vi "Validate Path.vi"(11 "Path in":path) -> (3 "Path out":path)   [LabVIEW 2019, in "Panel.lvlib" / "Persistent Position.lvclass"]
doc: "Checks a path for validity. If the input path is not valid, a default valid path will be generated.\n\n----\nPlease see the following web address for additional documentation and tutorial information:\nhttp://www.mooregoodideas.com/mgi-panel-manager/\n\nAuthor: Derek Trepanier\n\nCopyright (c) 2018, Moore Good Ideas, Inc.\n\nAll rights reserved.\n\nRedistribution and use in source and binary forms, with or without modification, are permitted provided that the following conditions are met:\n\n * Redistributions of source code must retain the above copyright notice, this list of conditions and the following disclaimer.\n * Redistributions in binary form must reproduce the above copyright notice, this list of conditions and the following disclaimer in the documentation and/or other materials provided with the distribution.\n * Neither the name of Moore Good Ideas, Inc. nor the names of its contributors may be used to endorse or promote products derived from this software without specific prior written permission.\n\nTHIS SOFTWARE IS PROVIDED BY THE COPYRIGHT HOLDERS AND CONTRIBUTORS \"AS IS\" AND ANY EXPRESS OR IMPLIED WARRANTIES, INCLUDING, BUT NOT LIMITED TO, THE IMPLIED WARRANTIES OF MERCHANTABILITY AND FITNESS FOR A PARTICULAR PURPOSE ARE DISCLAIMED. IN NO EVENT SHALL THE COPYRIGHT OWNER OR CONTRIBUTORS BE LIABLE FOR ANY DIRECT, INDIRECT, INCIDENTAL, SPECIAL, EXEMPLARY, OR CONSEQUENTIAL DAMAGES (INCLUDING, BUT NOT LIMITED TO, PROCUREMENT OF SUBSTITUTE GOODS OR SERVICES; LOSS OF USE, DATA, OR PROFITS; OR BUSINESS INTERRUPTION) HOWEVER CAUSED AND ON ANY THEORY OF LIABILITY, WHETHER IN CONTRACT, STRICT LIABILITY, OR TORT (INCLUDING NEGLIGENCE OR OTHERWISE) ARISING IN ANY WAY OUT OF THE USE OF THIS SOFTWARE, EVEN IF ADVISED OF THE POSSIBILITY OF SUCH DAMAGE."
uses:
  Persistent Position.lvclass
  <vilib>/Utility/sysdir.llb/System Directory Type.ctl
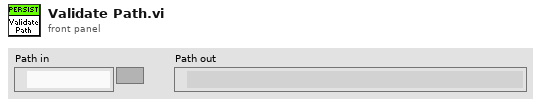
[diagram p1: front panel]
types:
  T1 = typedef "System Directory Type.ctl" = i32
  T2 = enum32{"invalid app kind", "Development System", "Run Time System", "Student Edition", "Embedded LabVIEW", "Evaluation", "Custom"}
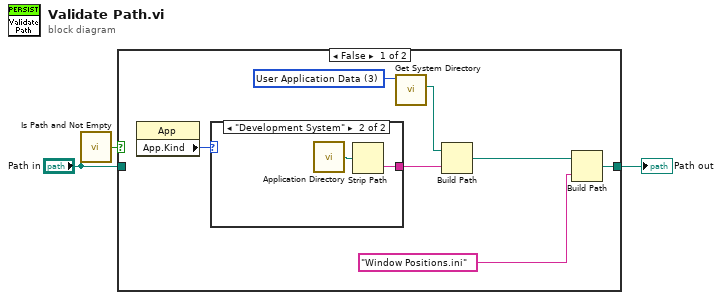
[diagram p0: block diagram]
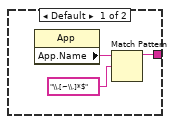
[diagram p2: hidden frame]
diagram:
  n1 = call <vilib>:"Is Path and Not Empty.vi"("path"="Path in") -> ("Is Path and Not Empty?"=w1:bool)  [unwired: 4 in]
  n2 = case shown="False" w1 {
    tunnel: "Path in" -> [_ w16]
    tunnel: [w5 w16] -> w3
    frame False {
      w10 = T1 3 items=["User Home"=0, "User Desktop"=1, "User Documents"=2, "User Application Data"=3, "User Preferences"=4, "User Temporary"=5, "Public Documents"=6, "Public Application Data"=7, "Public Preferences"=8, "Public Cache"=13, "System Core Libraries"=9, "System Installed Libraries"=10, "Application Files"=11, "Boot Volume Root"=12] ("system directory type")
      n3 = property class="App"() -> ("App.Kind"=w9:T2)  [unwired: 2 in, 2 out]
      n4 = case shown="\"Development System\"" w9 {
        tunnel: [w11 w14] -> w7
        frame Default {
          n5 = property class="App"() -> ("App.Name"=w13:string)  [unwired: 2 in, 2 out]
          n6 = Match Pattern(string=w13, regular expression="\\.[~\\.]*$") -> (before substring=w11:string)  [unwired: 1 in, 3 out]
        }
        frame "Development System" {
          n7 = call <vilib>:"Application Directory.vi"() -> ("Application Directory"=w15:path)
          n8 = Strip Path(path=w15) -> (name=w14:string)  [unwired: 1 out]
        }
      }
      n9 = call <vilib>:"Get System Directory.vi"("system directory type"=w10) -> ("system directory"=w8:path)  [unwired: 10 in]
      n10 = Build Path(base path=w8, name or relative path=w7) -> (appended path=w4:path)
      n11 = Build Path(base path=w4, name or relative path="Window Positions.ini") -> (appended path=w5:path)
    }
    frame True {
    }
  }
  "Path out" <- w3
